vi "Get Min-Max Encoder Limits.vi"() -> (0 "MinEncoder(in.)":dbl, 1 "MaxEncoder(in.)":dbl, 2 "MinEncoder":i32, 3 "MaxEncoder":i32)   [LabVIEW 2015, in "Tool Cfg.lvlib"]
uses:
  Tool Cfg.lvlib
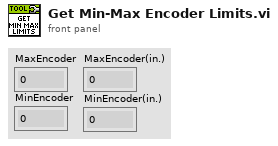
[diagram p1: front panel]
types:
  T1 = typedef "Tool Cfg.lvlib/_Tool Block Cluster_v3--typedef.ctl" = cluster{"Encoder Size":u16, "Encoder Scale":u32, "Encoder Offset":i32, "MaxEncoder":i32, "MinEncoder":i32, "Start Delay":sgl, "Tool Face Ref":sgl}
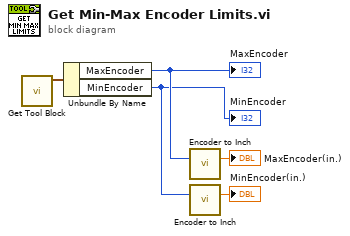
[diagram p0: block diagram]
diagram:
  n1 = call "Get Tool Block.vi"() -> ("Tool Block"=w5:T1)  [unwired: 11 in]
  n2 = Unbundle By Name(w5) -> ("MaxEncoder"=w4:i32, "MinEncoder"=w3:i32)
  "MaxEncoder" <- w4
  "MinEncoder" <- w3
  n3 = call "Encoder to Inch.vi"("Encoder in"=w4) -> ("Encoder out(in)"=→"MaxEncoder(in.)":dbl)  [unwired: 14 in]
  n4 = call "Encoder to Inch.vi"("Encoder in"=w3) -> ("Encoder out(in)"=→"MinEncoder(in.)":dbl)  [unwired: 14 in]
